vi "Get Variant Property.vi"(8 "error in (no error)":errorcluster, 9 "Histogram Graph Reference":refnum<vi>, 10 "Selected Item":string, 11 ".NET Refnum in":refnum<k24>) -> (0 "error out":errorcluster, 2 "Cluster":T1, 3 ".NET Refnum out":refnum<k24>)   [LabVIEW 2012]
uses:
  NationalInstruments.VeriStand.SystemStorage
  NationalInstruments.VeriStand
  <vilib>/NI Veristand/Custom Device Offline API/Custom Device Offline API.lvlib
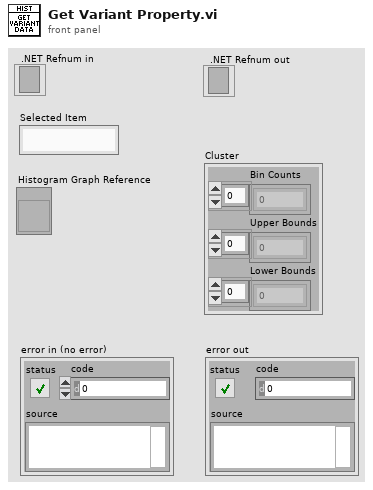
[diagram p1: front panel]
types:
  T1 = cluster{"Bin Counts":i32[], "Upper Bounds":dbl[], "Lower Bounds":dbl[]}
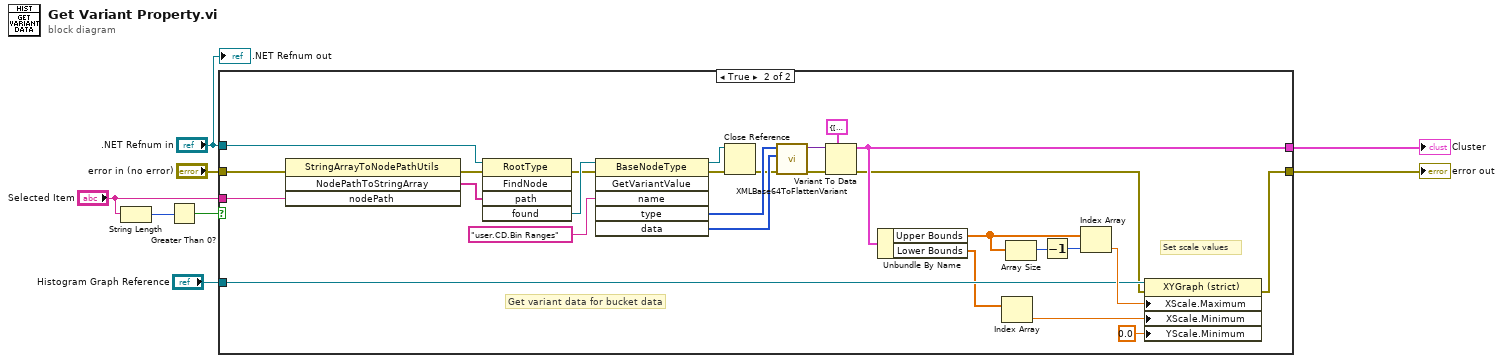
[diagram p0: block diagram]
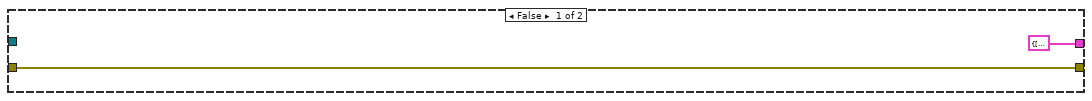
[diagram p2: hidden frame]
diagram:
  n1 = String Length(string="Selected Item") -> (length=w3:i32)
  n2 = Greater Than 0?(x=w3) -> (x > 0?=w4:bool)
  n3 = case shown="True" w4 {
    tunnel: "Selected Item" -> [_ w37]
    tunnel: ".NET Refnum in" -> [_ w35]
    tunnel: [T1 {"Bin Counts"=[], "Upper Bounds"=[], "Lower Bounds"=[]} ("Cluster") w16] -> w6
    tunnel: [w9 w12] -> w7
    tunnel: "error in (no error)" -> [w9 w22]
    tunnel: "Histogram Graph Reference" -> [_ w17]
    frame False {
    }
    frame True {
      # "Set scale values"
      # "Get variant data for bucket data"
      n4 = invoke class="StringArrayToNodePathUtils" method="NodePathToStringArray"(error in=w22, "nodePath"=w37) -> (error out=w34:errorcluster, "NodePathToStringArray"=w36:string[])  [unwired: 2 in, 2 out]
      n5 = invoke class="RootType" method="FindNode"(reference=w35, error in=w34, "path"=w36) -> (error out=w23:errorcluster, "found"=w32:refnum<k24>)  [unwired: 2 in, 3 out]
      n6 = invoke class="BaseNodeType" method="GetVariantValue"(reference=w32, error in=w23, "name"="user.CD.Bin Ranges") -> (reference out=w27:refnum<k24>, error out=w26:errorcluster, "type"=w31:u8[], "data"=w30:u8[])  [unwired: 3 in, 2 out]
      n7 = Close Reference(reference=w27, error in (no error)=w26) -> (error out=w25:errorcluster)
      n8 = call <vilib>:"XMLBase64ToFlattenVariant.vi"("error in (no error)"=w25, "Data"=w30, "Type array"=w31) -> ("error out"=w24:errorcluster, "Variant"=w29:variant)  [unwired: 7 in]
      n9 = Variant To Data(error in=w24, type=T1 {"Bin Counts"=[], "Upper Bounds"=[], "Lower Bounds"=[]} ("Cluster"), Variant=w29) -> (data=w16:T1, error out=w13:errorcluster)
      n10 = Unbundle By Name(w16) -> ("Upper Bounds"=w15:dbl[], "Lower Bounds"=w14:dbl[])
      n11 = Index Array(array=w14) -> (element=w21:dbl)  [unwired: 1 in]
      n12 = Array Size(array=w15) -> (size(s)=w20:i32)
      n13 = Decrement(x=w20) -> (x-1=w19:i32)
      n14 = Index Array(array=w15, index=w19) -> (element=w18:dbl)
      n15 = property on="Property Node" class="XYGraph (strict)"(reference=w17, error in=w13, "XScale.Maximum"=w18, "XScale.Minimum"=w21, "YScale.Minimum"=0.0 ("Y Scale.Range:Minimum")) -> (error out=w12:errorcluster)  [unwired: 1 out]
    }
  }
  "error out" <- w7
  "Cluster" <- w6
  ".NET Refnum out" <- ".NET Refnum in"
